vi "Get file.vi"(8 "error in (no error)":errorcluster, 9 "Local path":path, 10 "Remote path":string, 11 "WebDAV in":refnum<class "WebDAV.lvclass">) -> (0 "error out":errorcluster, 3 "WebDAV out":refnum<class "WebDAV.lvclass">)   [LabVIEW 2015, in "RT Management.lvlib" / "WebDAV.lvclass"]
uses:
  WebDAV.lvclass
  WebDAV.lvclass/WebDAV.ctl
  Get Session.vi
  <vilib>/WebDAVClient/Advanced/Get File.vi
  <vilib>/WebDAVClient/NI_WebDAV.lvlib
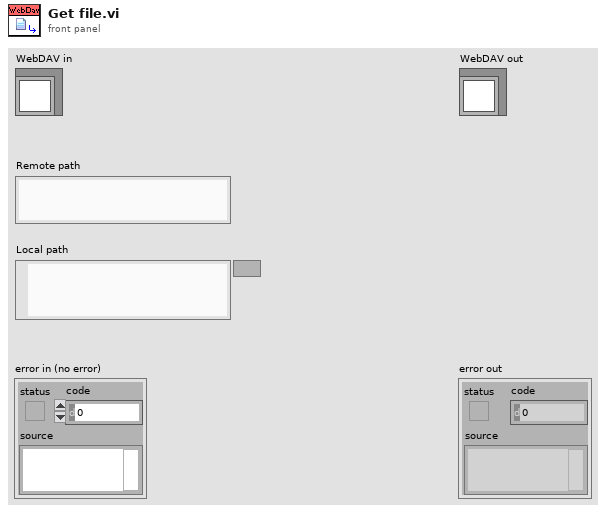
[diagram p1: front panel]
types:
  T1 = typedef "NI_WebDAV.lvlib/SessionHandle.ctl" = refnum<k1>
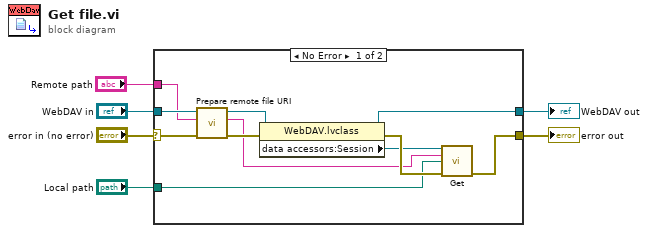
[diagram p0: block diagram]
diagram:
  n1 = case shown="No Error" "error in (no error)" {
    selector: "error in (no error)" -> [w9 w19]
    tunnel: [w17 w19] -> w5
    tunnel: "WebDAV in" -> [w10 w18]
    tunnel: [w16 w18] -> w3
    tunnel: "Remote path" -> [w8 _]
    tunnel: "Local path" -> [w7 _]
    frame No Error {
      n2 = call "Prepare remote file URI.vi"("error in (no error)"=w9, "Remote path"=w8, "WebDAV in"=w10) -> ("error out"=w13:errorcluster, "Remote file URI"=w11:string, "WebDAV out"=w12:refnum<class "WebDAV.lvclass">)  [unwired: 6 in]
      n3 = property class="WebDAV.lvclass"(reference=w12, error in=w13) -> (reference out=w16:refnum<class "WebDAV.lvclass">, error out=w15:errorcluster, "data accessors:Session"=w14:T1)
      n4 = call-poly <vilib>:"Get.vi"("session handle"=w14, "relative uri"=w11, "local file path"=w7, "error in (no error)"=w15) -> ("error out"=w17:errorcluster)  [unwired: 9 in, 2 out]
    }
    frame Error {
    }
  }
  "error out" <- w5
  "WebDAV out" <- w3
